vi "vision_webcam_V3.vi"(11 "dup Message Queue 2":refnum<queue>) -> ()   [LabVIEW 2017]
uses:
  UI Error Handlers/support/Message Queue/Message Cluster.ctl
  <vilib>/vision/Image Controls.llb/IMAQ Image.ctl
  camera_array_1.ctl
  <vilib>/userdefined/High Color/IMAQdx.ctl
  Globals/Global - Configuration Options.vi
  Globals/Global - All RT Loop Stop.vi
  <vilib>/vision/driver/NI_Vision_Acquisition_Software.lvlib
  UI Error Handlers/support/Message Queue/Message Queue.lvlib
panel:
  out "Images":T1
  out "Array":T2[](array[typedef])
  out "x-y":u32
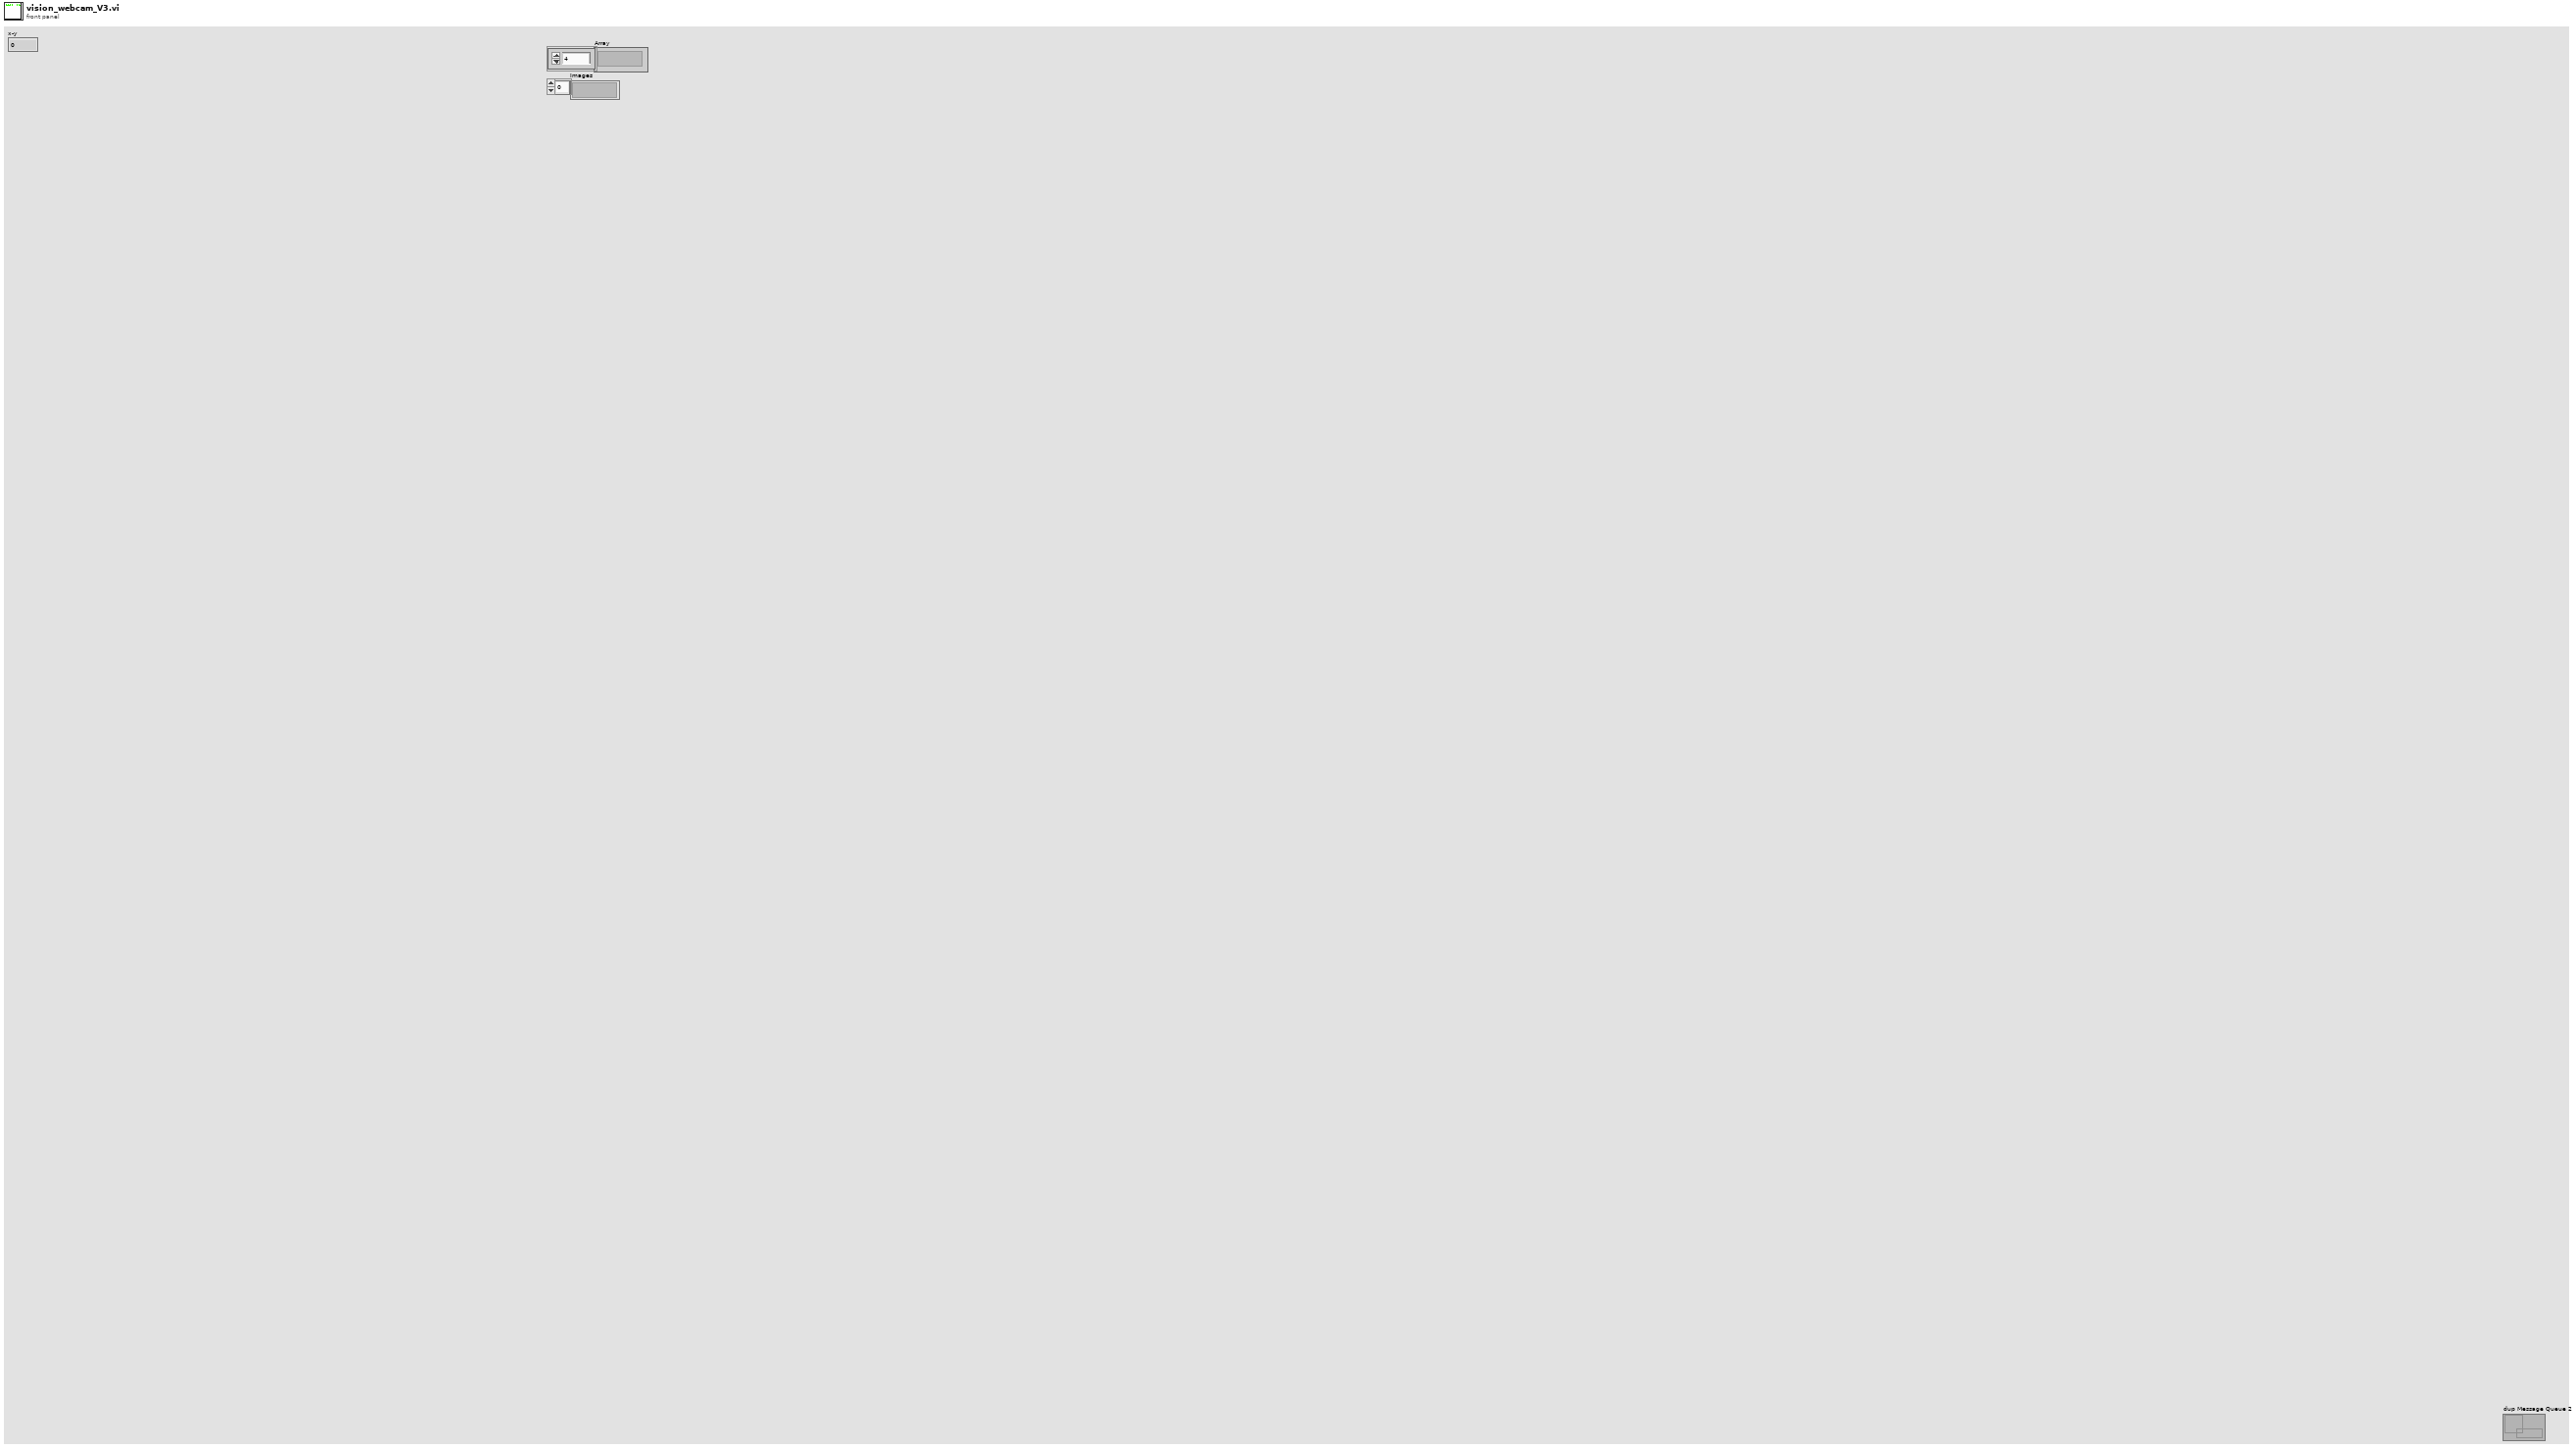
[diagram p1: front panel]
types:
  T1 = typedef "camera_array_1.ctl" = T2[]
  T2 = typedef "IMAQ Image.ctl" = refnum<image>
  T3 = typedef "IMAQdx.ctl" = refnum<k21>
  T4 = typedef "Image Type" = u32
  T5 = cluster{"Tool data":cluster{"Number of teeth":sgl}, "Cutting data":cluster{"rpm":sgl}, "Limits":cluster{"Magnitude threshold":sgl, "Tolerance":sgl}, "G1 status":cluster{"G1 trigger":bool}}
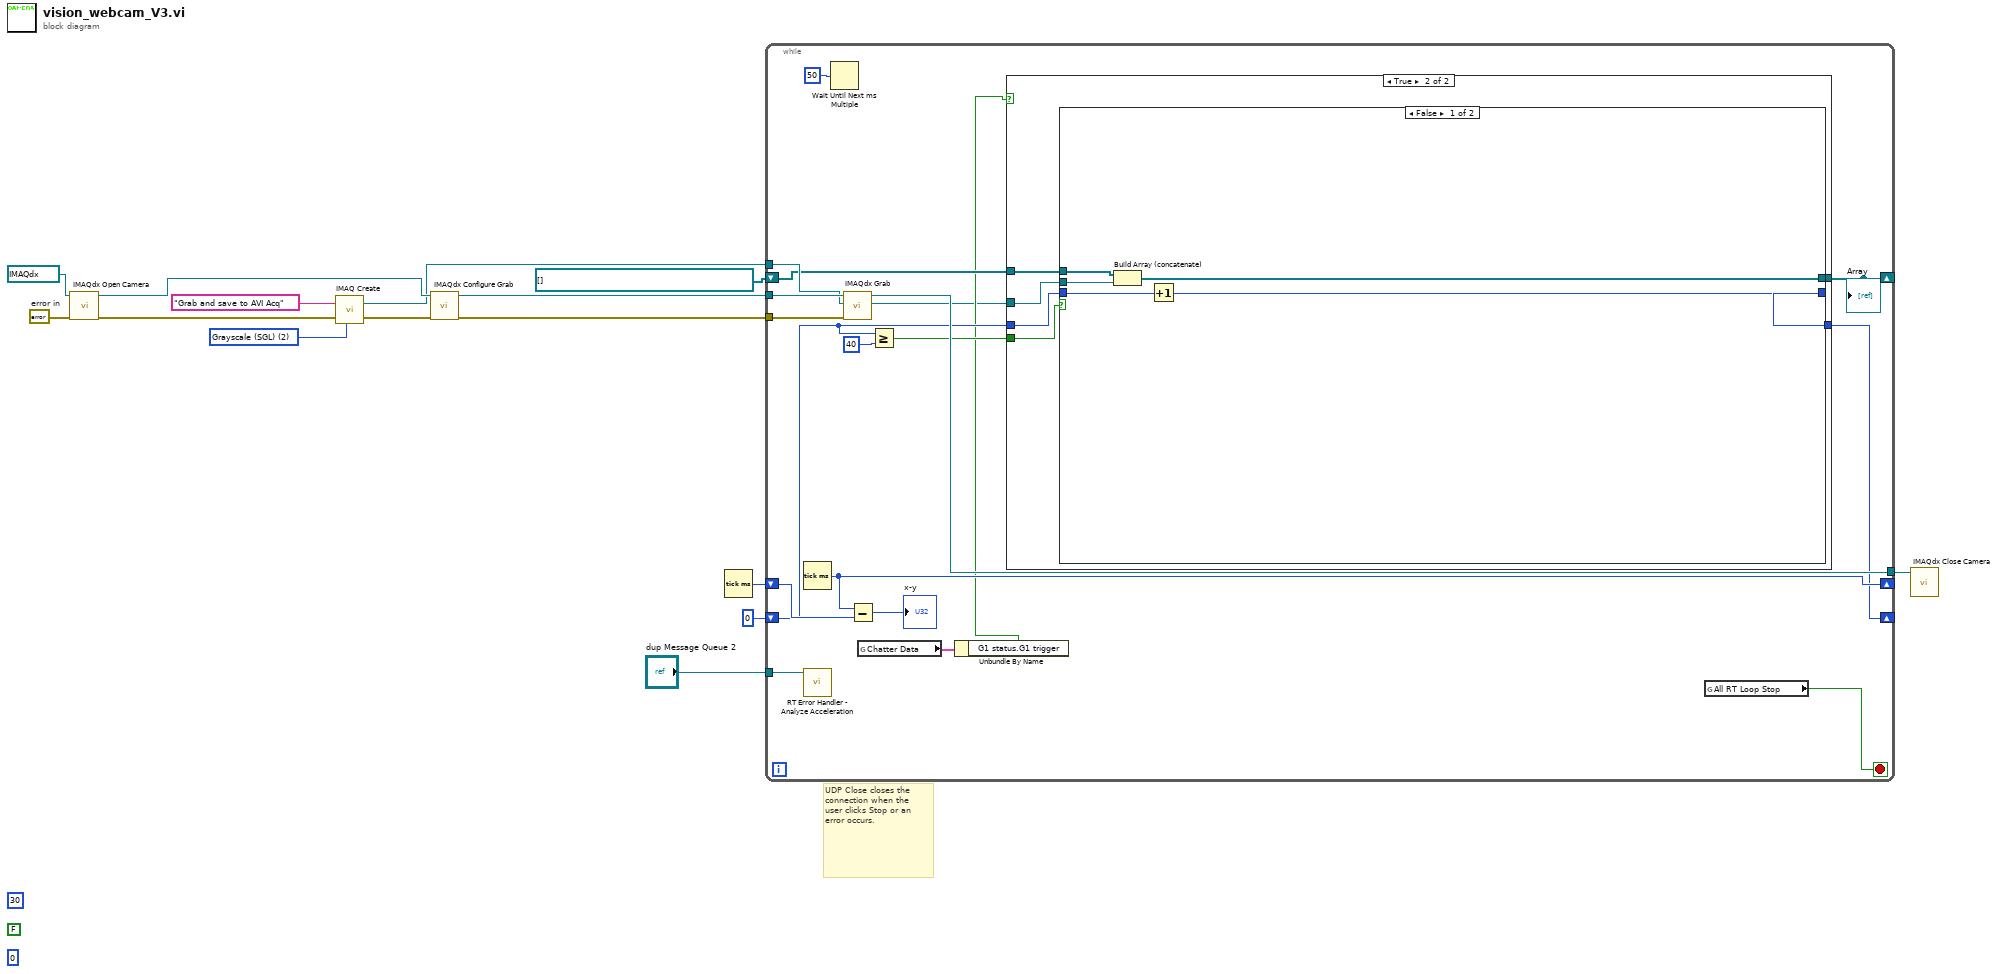
[diagram p0: block diagram]
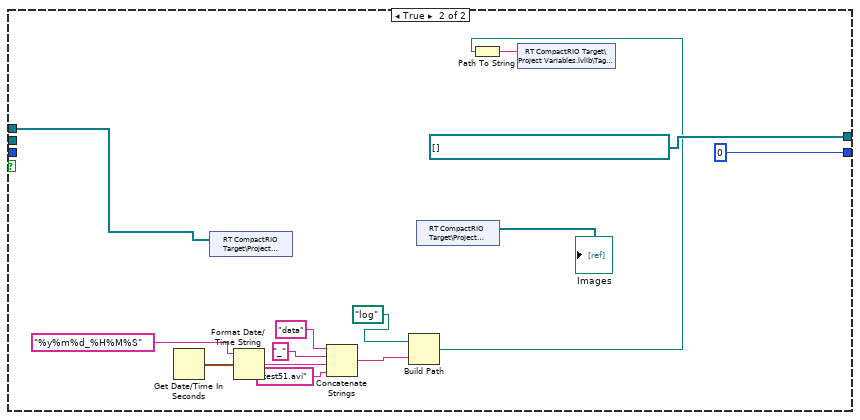
[diagram p3: hidden frame]
diagram:
  w10 = T4 2 items=["Grayscale (U8)", "Grayscale (I16)", "Grayscale (SGL)", "Complex (CSG)", "RGB (U32)", "HSL (U32)", "RGB (U64)", "Grayscale (U16)"] ("Image Type")
  (unwired) u32 30 ("Frames Per Second")
  w11 = errorcluster {"status"=FALSE, "code"=0, "source"=""}  # error in
  (unwired) i16 0 ("A(I16) 11")
  (unwired) FALSE
  # "UDP Close closes the connection when the user clicks Stop or an error occurs."
  n1 = call <vilib>:"IMAQdx Open Camera.vi"("error in"=w11, "Session In"=T3 "cam0") -> ("error out"=w9:errorcluster, "Session Out"=w13:T3)  [unwired: 8 in]
  n2 = call "IMAQ Create"("Image Name"="Grab and save to AVI Acq", "Image Type"=w10, "error in (no error)"=w9) -> ("New Image"=w6:T2, "error out"=w5:errorcluster)  [unwired: 2 in]
  n3 = call <vilib>:"IMAQdx Configure Grab.vi"("error in"=w5, "Session In"=w13) -> ("error out"=w4:errorcluster, "Session Out"=w7:T3)  [unwired: 8 in]
  n4 = Tick Count (ms)() -> (millisecond timer value=w14:u32)
  n5 = while {
    tunnel: "dup Message Queue 2" -> [w34]
    shift-right: [w30] -> _
    shift-left: w14 -> [w31]
    tunnel: w7 -> [w29]
    tunnel: w6 -> [w28]
    tunnel: w4 -> [w27]
    tunnel: [w26] -> w3
    shift-right: [w19] -> _
    shift-left: T2[] [] -> [w23]
    shift-right: [w20] -> _
    shift-left: 0 -> [w21]
    stop <- w18 stop-if-true
    n6 = Tick Count (ms)() -> (millisecond timer value=w30:u32)
    n7 = call "RT Error Handler - Analyze Acceleration.vi"("Message Queue"=w34) -> ()  [unwired: 10 in, 1 out]
    n8 = Wait Until Next ms Multiple(millisecond multiple=u32 50) -> ()  [unwired: 1 out]
    n9 = call <vilib>:"IMAQdx Grab.vi"("error in"=w27, "Image In"=w28, "Session In"=w29) -> ("Image Out"=w16:T2, "Session Out"=w26:T3)  [unwired: 5 in, 2 out]
    n10 = Subtract(x=w30, y=w31) -> (x-y=→"x-y":u32)
    n11 = global read "Global - Configuration Options.vi" "Chatter Data"() -> (w33:T5)
    n12 = Greater Or Equal?(x=w21, y=40) -> (x >= y?=w22:bool)
    n13 = Unbundle By Name(w33) -> ("G1 status.G1 trigger"=w17:bool)
    n14 = case shown="True" w17 {
      tunnel: w16 -> [_ w42]
      tunnel: w23 -> [w35 w40]
      tunnel: w22 -> [_ w41]
      tunnel: w21 -> [w36 w39]
      tunnel: [w36 w38] -> w20
      tunnel: [w35 w37] -> w19
      frame False {
      }
      frame True {
        n15 = case shown="False" w41 {
          tunnel: w42 -> [w46 _]
          tunnel: w40 -> [w47 w58]
          tunnel: w39 -> [w45 _]
          tunnel: [w44 0] -> w38
          tunnel: [w43 T2[] []] -> w37
          frame False {
            n16 = Build Array (concatenate)(w47, w46) -> (w43:T2[])
            n17 = Increment(x=w45) -> (x+1=w44:i32)
          }
          frame True {
            n18 = Get Date/Time In Seconds() -> (seconds since 1Jan1904=w55:timestamp)
            n19 = shared-variable "RT CompactRIO Target\\Project Variables.lvlib\\Images"(w58) -> ()  [unwired: 1 in, 1 out]
            n20 = Format Date/Time String(time format string (%c)="%y%m%d_%H%M%S", seconds (now)=w55) -> (date/time string=w54:string)  [unwired: 1 out]
            n21 = Concatenate Strings("data" ("string"), "_" ("string"), w54, "test51.avi" ("string")) -> (w56:string)
            n22 = Build Path(base path=path "log", name or relative path=w56) -> (appended path=w48:path)
            n23 = shared-variable "RT CompactRIO Target\\Project Variables.lvlib\\Images"() -> (→"Images":T1)  [unwired: 1 in, 1 out]
            n24 = Path To String(path=w48) -> (string=w61:string)
            n25 = shared-variable "RT CompactRIO Target\\Project Variables.lvlib\\Tag Video"(w61) -> ()  [unwired: 1 in, 1 out]
          }
        }
      }
    }
    "Array" <- w19
    n26 = global read "Global - All RT Loop Stop.vi" "All RT Loop Stop"() -> (w18:bool)
  }
  n27 = call <vilib>:"IMAQdx Close Camera.vi"("Session In"=w3) -> ()  [unwired: 10 in, 1 out]
